vi "InitializeSessions.vi"(0 "Keysight_34401A-DMM in":refnum<class "Keysight_34401A-DMM.lvclass">, 5 "InitializeSessionsInfo":variant, 11 "error in (no error)":errorcluster) -> (4 "Keysight_34401A-DMM out":refnum<class "Keysight_34401A-DMM.lvclass">, 15 "error out":errorcluster)   [LabVIEW 2020, in "Keysight_34401A-DMM.lvclass"]
uses:
  Keysight_34401A-DMM.lvclass
  C:/Program Files/National Instruments/LabVIEW 2020/vi.lib/MeasurementLink/MeasurementLink Instrument/ISession Factory/ISession Factory.lvclass
  TypeDef/Initialize_Information.ctl
  <vilib>/MeasurementLink/MeasurementLink Session Management V1/Session Reservation/Initialize and Close Session Behavior.ctl
  Keysight_34401A-DMM.lvclass/Keysight_34401A-DMM.ctl
  b116fd11-a7c2-4259-97aa-a06ad338d6e7.vi
  <vilib>/MeasurementLink/MeasurementLink Session Management V1/Session Reservation/Initialize Sessions with Retry.vi
  <vilib>/MeasurementLink/MeasurementLink Session Management V1/Session Reservation/Session Reservation.lvclass
panel:
  out "channel list":string
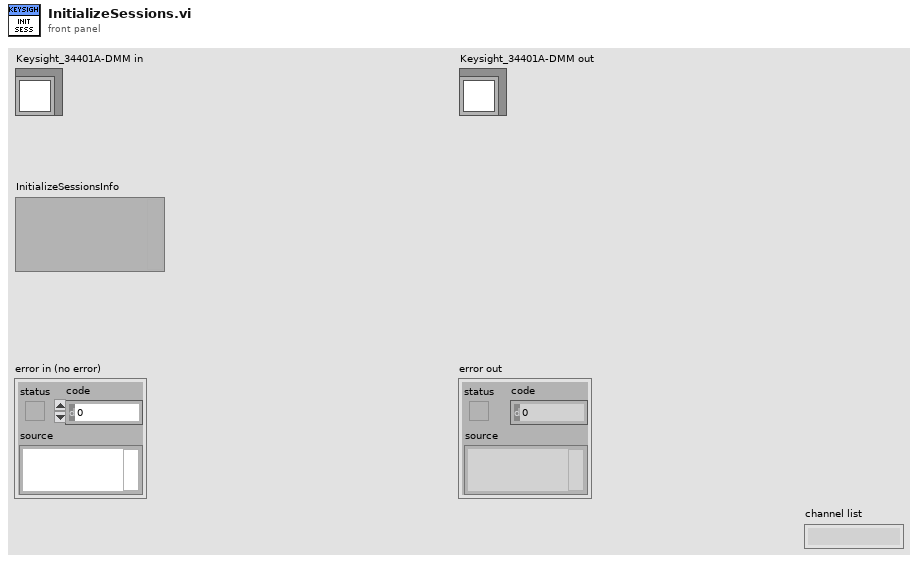
[diagram p1: front panel]
types:
  T1 = cluster{"Baud Rate":u32, "Parity":u16, "Data Bits":u16}
  T2 = typedef "Keysight_34401A-DMM.lvclass/Initialize_Information.ctl" = cluster{"initialize and close session behavior":T3, "reset":bool}
  T3 = typedef "MeasurementLink Session Management V1.lvlib/Session Reservation.lvclass/Initialize and Close Session Behavior.ctl" = enum16{"Auto", "Initialize and Close", "Attach and Detach", "Initialize and Detach", "Attach and Close"}
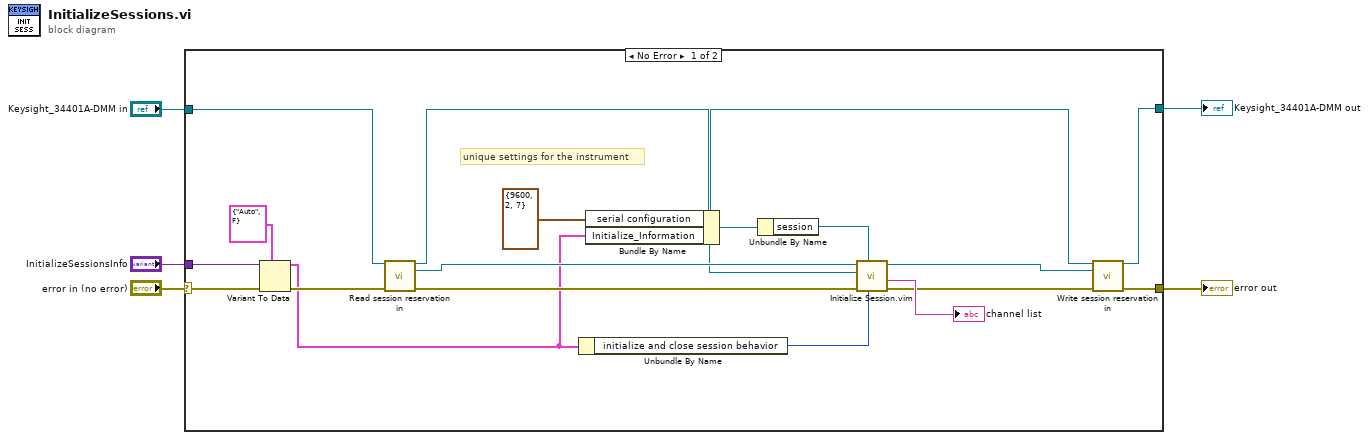
[diagram p0: block diagram]
diagram:
  n1 = case shown="No Error" "error in (no error)" {
    selector: "error in (no error)" -> [w22 w24]
    tunnel: "Keysight_34401A-DMM in" -> [w23 w25]
    tunnel: [w11 w24] -> w3
    tunnel: "InitializeSessionsInfo" -> [w20 _]
    tunnel: [w10 w25] -> w1
    frame No Error {
      # "unique settings for the instrument"
      n2 = Variant To Data(error in=w22, type=T2 {"initialize and close session behavior"=enum."Auto", "reset"=FALSE} ("Initialize_Information"), Variant=w20) -> (data=w6:T2, error out=w21:errorcluster)
      n3 = call-dynamic "Read session reservation in.vi"("AbstractDMM in"=w23, "error in (no error)"=w21) -> ("AbstractDMM out"=w19:refnum<class "Keysight_34401A-DMM.lvclass">, "MeasurementLink Session Management V1.lvlib:Session Reservation.lvclass"=w15:refnum<class "Session Reservation.lvclass">, "error out"=w16:errorcluster)  [unwired: 11 in]
      n4 = Unbundle By Name(w6) -> ("initialize and close session behavior"=w13:T3)
      n5 = Bundle By Name(cluster=w19, "serial configuration"=T1 {"Baud Rate"=9600, "Parity"=2, "Data Bits"=7}, "Initialize_Information"=w6) -> (w8:refnum<class "Keysight_34401A-DMM.lvclass">)
      n6 = Unbundle By Name(w8) -> ("session"=w7:refnum<visa-resource-name>)
      n7 = call "Initialize Session.vim"("initialize and close session behavior"=w13, "session type"=w7, "error in"=w16, "session factory"=w8, "session reservation in"=w15) -> ("error out"=w12:errorcluster, "channel list"=→"channel list":string, "session reservation out"=w9:refnum<class "Session Reservation.lvclass">)  [unwired: 3 in, 1 out]
      n8 = call-dynamic "Write session reservation in.vi"("AbstractDMM in"=w8, "MeasurementLink Session Management V1.lvlib:Session Reservation.lvclass"=w9, "error in (no error)"=w12) -> ("AbstractDMM out"=w10:refnum<class "Keysight_34401A-DMM.lvclass">, "error out"=w11:errorcluster)  [unwired: 11 in]
    }
    frame Error {
    }
  }
  "error out" <- w3
  "Keysight_34401A-DMM out" <- w1
